vi "Analysis_Result_To_Table_Value.vi"(9 "AnalysisResults":variant[](array[variant]), 11 "All ROI":T8[](array[typedef])) -> (2 "TableValues":string[](array[string]))   [LabVIEW 2019]
uses:
  Analysis/Controls/Parttern Match/Analysis_PatternMatch_Parameter.ctl
  Analysis/Controls/Edge Detection/Analysis_Edge Detection_Parameter.ctl
  Analysis/Controls/Barcode 1D/Analysis_Barcode 1D_Parameter.ctl
  <vilib>/vision/Instrument.llb/QR Code Model Type.ctl
  <vilib>/vision/Instrument.llb/Data Matrix Polarity.ctl
  <vilib>/vision/Instrument.llb/QR Code Description Options.ctl
  <vilib>/vision/Instrument.llb/Cell Filter Mode.ctl
  <vilib>/vision/Instrument.llb/Cell Sample Size.ctl
  <vilib>/vision/Instrument.llb/Demodulation Mode.ctl
  <vilib>/vision/Instrument.llb/QR Code Search Options.ctl
  Analysis/Controls/Barcode 2D/Analysis_Barcode 2D_Parameter.ctl
  Analysis/Controls/Clamp/Analysis_Clamp_Parameter.ctl
  Analysis/Controls/Clamp MAX/Analysis_Clamp MAX_Parameter.ctl
  Analysis/Controls/Particle/Analysis_Particle_Parameter.ctl
  Analysis/Controls/Find Straight Edge/Analysis_Find Straight Edge_Parameter.ctl
  <vilib>/vision/Measure.llb/Straight Edge Process.ctl
  <vilib>/vision/Measure.llb/Straight Edge Options.ctl
  <vilib>/vision/Measure.llb/Edge Polarity.ctl
  <vilib>/vision/Measure.llb/Edge Options.ctl
  <vilib>/vision/Instrument.llb/Data Matrix Search Options.ctl
  <vilib>/vision/Instrument.llb/Data Matrix Mirror.ctl
  <vilib>/vision/Instrument.llb/Cell Fill Percentage.ctl
  <vilib>/vision/Instrument.llb/ECC Type.ctl
  <vilib>/vision/Instrument.llb/Data Matrix Description Options.ctl
  Analysis/Controls/Histogram/Analysis_Histogram_Parameter.ctl
  Analysis/Controls/Circle/Analysis_Circle_Parameter.ctl
  Analysis/Controls/Parttern Match/Analysis_PatternMatch_ResultWithnumber.ctl
  Analysis/Controls/ShapeDectect/Analysis_ShapeDectect_Parameter.ctl
  Analysis/Controls/Contour/Analysis_Contour_Result.ctl
  Analysis/Controls/ColorMatch/Analysis_ColorMatch_Result.ctl
  <vilib>/vision/Instrument.llb/Data Matrix Advanced Options.ctl
  <vilib>/vision/Instrument.llb/Data Matrix Size Options.ctl
  Process/Controls/Process_Setting.ctl
  Analysis/Controls/Analysis_Setting.ctl
  Controls/Vision_DataEntry.ctl
  <vilib>/vision/Measure.llb/Edge New.ctl
  Analysis/Controls/V_Analysis_Type.ctl
  Ctrl/VisionProcessName.ctl
panel:
  in  "output cluster 2":T1
  in  "Particle Cluster":T2
  in  "output cluster":T3
  in  "Clamp Cluster":T4={"Points"=[], "Perpendicular Lines"=[], "appended array"=[], "Line Coordinates"=[], "Clamp Settings"={"Contrast"=0, "Filter width"=0, "Steepness"=0, "Subsampling Ratio"=0, "Show Search Area"=FALSE, "Show Search Lines"=FALSE, "Show Edges Found"=FALSE, "Show Result"=FALSE}, "ROI Descriptor"={"Global Rectangle"=[], "Contours"=[]}, "Distance"=0.0, "Edge Coordinates"=[{"X"=441.67966, "Y"=663.0}, {"X"=684.4586, "Y"=655.0}], "Edge Coordinates  (Real World)"=[{"X"=441.67966, "Y"=663.0}, {"X"=684.4586, "Y"=655.0}], "Distance (Real World)"=0.0}
  in  "Edge Detection Cluster":T6 {"Edge Information"."Distance (Real-World)" format="%.2f"; "Edge Information"."Location (Real-World)"."Y" format="%.2g"; "Edge Information"."Location (Real-World)"."X" format="%.2f"; "Edge Information"."Noise" format="%.2f"; "Edge Information"."Location (Pixel)"."Y" format="%.2g"; "Edge Information"."Location (Pixel)"."X" format="%.2f"; "Edge Information"."Strength" format="%.2f"; "Edge Information"."Distance (Pixel)" format="%.2f"}
  in  "Straight Edge Cluster Array":T7(array[cluster])
  in  "Barcode 2D Result cluster":T13
  in  "Barcode 1D output cluster":T14
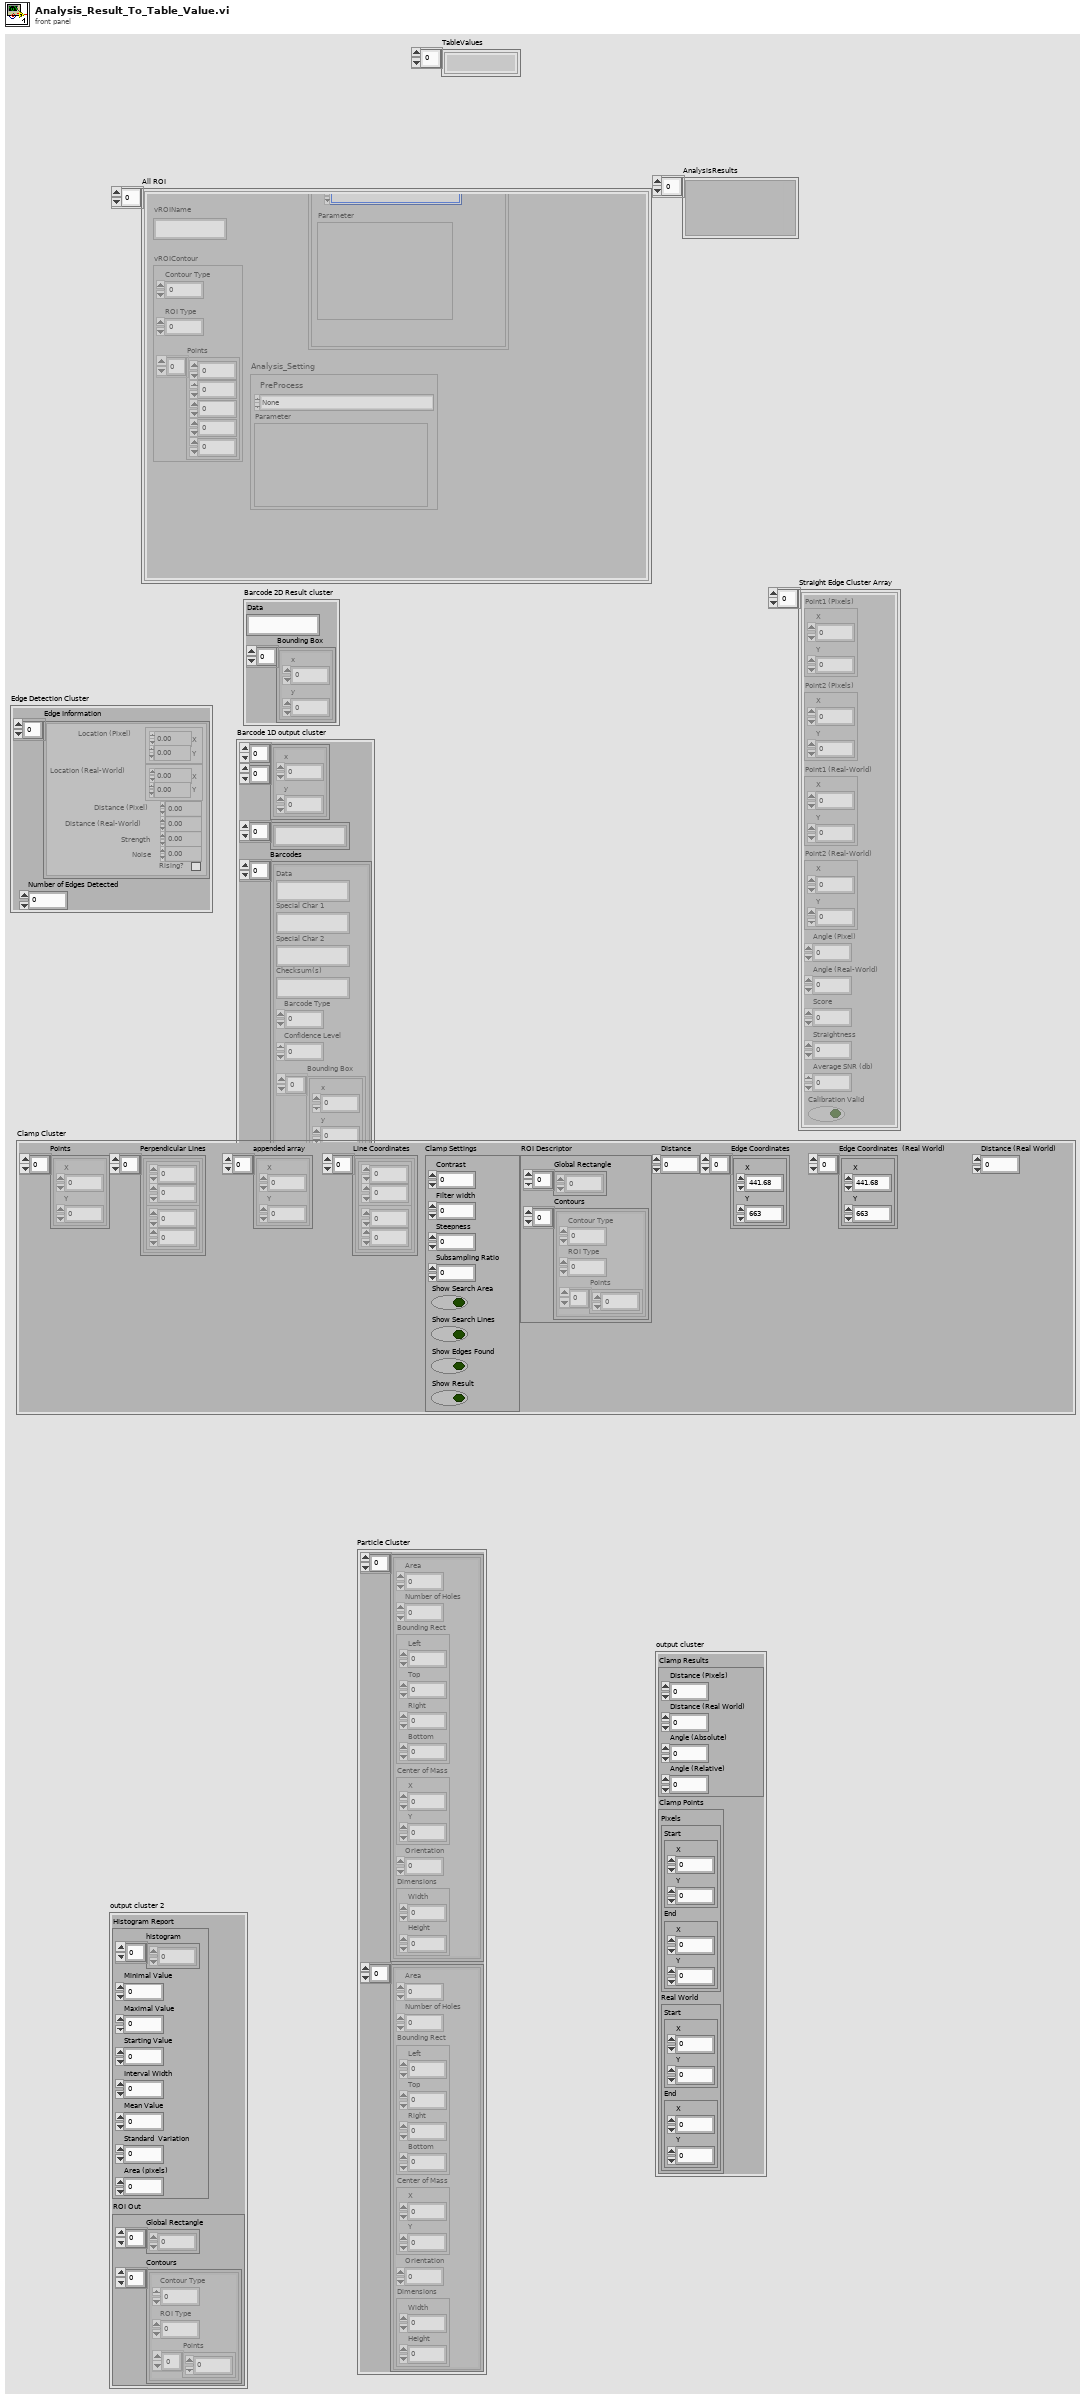
[diagram p1: front panel]
types:
  T1 = cluster{"Histogram Report":cluster{"histogram":u32[], "Minimal Value":sgl, "Maximal Value":sgl, "Starting Value":sgl, "Interval Width":sgl, "Mean Value":sgl, "Standard  Variation":sgl, "Area (pixels)":i32}, "ROI Out":cluster{"Global Rectangle":i32[], "Contours":cluster{"Contour Type":u32, "ROI Type":u32, "Points":i32[]}[]}}
  T2 = cluster{cluster{"Area":dbl, "Number of Holes":dbl, "Bounding Rect":cluster{"Left":dbl, "Top":dbl, "Right":dbl, "Bottom":dbl}, "Center of Mass":cluster{"X":dbl, "Y":dbl}, "Orientation":dbl, "Dimensions":cluster{"Width":dbl, "Height":dbl}}[], cluster{"Area":dbl, "Number of Holes":dbl, "Bounding Rect":cluster{"Left":dbl, "Top":dbl, "Right":dbl, "Bottom":dbl}, "Center of Mass":cluster{"X":dbl, "Y":dbl}, "Orientation":dbl, "Dimensions":cluster{"Width":dbl, "Height":dbl}}[]}
  T3 = cluster{"Clamp Results":cluster{"Distance (Pixels)":dbl, "Distance (Real World)":dbl, "Angle (Absolute)":dbl, "Angle (Relative)":dbl}, "Clamp Points":cluster{"Pixels ":cluster{"Start":cluster{"X":dbl, "Y":dbl}, "End":cluster{"X":dbl, "Y":dbl}}, "Real World":cluster{"Start":cluster{"X":dbl, "Y":dbl}, "End":cluster{"X":dbl, "Y":dbl}}}}
  T4 = cluster{"Points":cluster{"X":sgl, "Y":sgl}[], "Perpendicular Lines":cluster{cluster{sgl, sgl}, cluster{sgl, sgl}}[], "appended array":cluster{"X":sgl, "Y":sgl}[], "Line Coordinates":cluster{cluster{sgl, sgl}, cluster{sgl, sgl}}[], "Clamp Settings":cluster{"Contrast":i32, "Filter width":i32, "Steepness":i32, "Subsampling Ratio":u32, "Show Search Area":bool, "Show Search Lines":bool, "Show Edges Found":bool, "Show Result":bool}, "ROI Descriptor":cluster{"Global Rectangle":i32[], "Contours":cluster{"Contour Type":u32, "ROI Type":u32, "Points":i32[]}[]}, "Distance":sgl, "Edge Coordinates":cluster{"X":sgl, "Y":sgl}[], "Edge Coordinates  (Real World)":cluster{"X":sgl, "Y":sgl}[], "Distance (Real World)":sgl}
  T5 = typedef "Edge New.ctl" = cluster{"Location (Pixel)":cluster{"X":sgl, "Y":sgl}, "Location (Real-World)":cluster{"X":sgl, "Y":sgl}, "Distance (Pixel)":dbl, "Distance (Real-World)":dbl, "Strength":dbl, "Noise":dbl, "Rising?":bool}
  T6 = cluster{"Edge Information":T5[], "Number of Edges Detected":i32}
  T7 = cluster{"Point1 (Pixels)":cluster{"X":sgl, "Y":sgl}, "Point2 (Pixels)":cluster{"X":sgl, "Y":sgl}, "Point1 (Real-World)":cluster{"X":sgl, "Y":sgl}, "Point2 (Real-World)":cluster{"X":sgl, "Y":sgl}, "Angle (Pixel)":dbl, "Angle (Real-World)":dbl, "Score":dbl, "Straightness":dbl, "Average SNR (db)":dbl, "Calibration Valid":bool}[]
  T8 = typedef "Vision_DataEntry.ctl" = cluster{"vROIName":string, "vROIContour":cluster{"Contour Type":u32, "ROI Type":u32, "Points":i32[]}, "ProcessSetting":T9[], "Analysis_Setting":T11}
  T9 = typedef "Process_Setting.ctl" = cluster{"Enum_PreProcess":T10, "Parameter":string}
  T10 = typedef "VisionProcessName.ctl" = enum16{"*CamParameter*", "CamAttributes", "*Preprocess*", "CG_Brightness", "C_Plane Extraction", "C_Threshold", "G_Lookup Table", "G_Threshold"}
  T11 = typedef "Analysis_Setting.ctl" = cluster{"PreProcess":T12, "Parameter":string}
  T12 = typedef "V_Analysis_Type.ctl" = enum16{"None", "C_Color Pattern Matching", "G_PatternMatching", "G_ShapeDectect", "G_GeometricMatch", "B_Area Check"}
  T13 = cluster{"Data":string, "Bounding Box":cluster{"x":sgl, "y":sgl}[]}
  T14 = cluster{cluster{"x":sgl, "y":sgl}[][], string[], "Barcodes":cluster{"Data":string, "Special Char 1":string, "Special Char 2":string, "Checksum(s)":string, "Barcode Type":u32, "Confidence Level":sgl, "Bounding Box":cluster{"x":sgl, "y":sgl}[]}[]}
  T15 = typedef "ROI Descriptor" = cluster{"Global Rectangle":i32[], "Contours":cluster{"ID":enum32{"External", "Internal"}, "Type":u32, "Coordinates":i32[]}[]}
  T16 = cluster{"Algorithm":i32, "Match Parameters":cluster{"Number of Matches Requested":i32, "Minimum Match Score":sgl, "Angle Ranges":cluster{"Start Angle":sgl, "End Angle":sgl}[]}, "ROI Descriptor":T15, "Advanced Options":cluster{"Item":u16, "Value":dbl}[], "Template path":string}
  T17 = typedef "Analysis_Histogram_Parameter.ctl" = cluster{"Interval Range":cluster{"Minimum":sgl, "Maximum":sgl}, "ROI Out":cluster{"Global Rectangle":i32[], "Contours":cluster{"Contour Type":u32, "ROI Type":u32, "Points":i32[]}[]}, "Number of Classes":i32}
  T18 = cluster{"ROI Descriptor out":T15, "ROI Descriptor out":T15, "Fitted Circle":cluster{"Center (Pixels)":cluster{"X":sgl, "Y":sgl}, "Radius (Pixels)":dbl, "Center (Real-World)":cluster{"X":sgl, "Y":sgl}, "Radius (Real-World)":dbl, "Roundness (Real-World)":dbl, "Average Strength":dbl, "Average SNR (dB)":dbl}}
  T19 = typedef "Analysis_ShapeDectect_Parameter.ctl" = cluster{"Enum_ShapeType":enum16{"Circles", "Ellipses", "Lines", "Rectangles"}, "MaxParticle":i32, "Descriptor":cluster{"Set 1":dbl, "Set 2":dbl, "Set 3":dbl, "Set 4":dbl}, "Match Options":cluster{"Rotation":bool, "Scale":bool, "Occlusion":bool, "Range Settings":cluster{"Match Constraints":u32, "Min":dbl, "Max":dbl}[]}, "Curve Parameters":cluster{"Extraction Mode":u32, "Edge Threshold":i32, "Edge Filter Size":u32, "Min Length":i32, "Row Search Step Size":i32, "Col Search Step Size":i32, "Max Endpoint Gap":i32, "Closed":bool, "Subpixel":bool}, " score":dbl}
  T20 = typedef "Analysis_Contour_Result.ctl" = cluster{"Points (pixel)":cluster{"X":dbl, "Y":dbl}[], "Points (real)":cluster{"X":dbl, "Y":dbl}[], "Length (pixel)":dbl, "Length (real)":dbl}
  T21 = typedef "Analysis_ColorMatch_Result.ctl" = cluster{"Match Flag":bool[], "Match Score":i32[], "ROI Descriptor":T15}
  T22 = typedef "Analysis_Type.ctl" = u16
  T23 = typedef "Analysis_PatternMatch_ResultWithnumber.ctl" = cluster{"numbers":i32, "results":cluster{"ROI Descriptor out":T15, "Point":T24, "Angle":sgl, "Score":sgl, "Real World Coordinates":cluster{"X":sgl, "Y":sgl}, "Rectangle":T25}[]}
  T24 = typedef "IMAQ Point" = cluster{"X":sgl, "Y":sgl}
  T25 = typedef "IMAQ Rectangle" = cluster{"Left":i32, "Top":i32, "Right":i32, "Bottom":i32, "Rotation":dbl}
  T26 = typedef "Analysis_PatternMatch_Parameter.ctl" = cluster{"Algorithm":i32, "Match Parameters":cluster{"Number of Matches Requested":i32, "Minimum Match Score":sgl, "Angle Ranges":cluster{"Start Angle":sgl, "End Angle":sgl}[]}, "ROI Descriptor":T15, "Advanced Options":cluster{"Item":u16, "Value":dbl}[], "Template path":string, "XOffset":i32, "YOffset":i32}
  T27 = cluster{"Number of Matches Requested":i32, "Minimum Match Score":sgl, "Angle Ranges":cluster{"Start Angle":sgl, "End Angle":sgl}[]}
  T28 = typedef "Analysis_Edge Detection_Parameter.ctl" = cluster{"Edge Options":cluster{"Edge Polarity":u16, "Kernel Size":u32, "Width":u32, "Minimum Edge Strength":dbl, "Interpolation Type":u16, "Data Processing Method":u16}, "Process":u16, "Number of Matches Requested":i32, "ROI Descriptor":cluster{"Global Rectangle":i32[], "Contours":cluster{"Contour Type":u32, "ROI Type":u32, "Points":i32[]}[]}}
  T29 = typedef "Analysis_Barcode 1D_Parameter.ctl" = cluster{"Barcode Search Options":cluster{"Min Bar Width":dbl, "Min Edge Strength":dbl, "Min Bars":dbl, "Skip Location Search?":bool}, "Barcode Types To Search":enum16{"Reserved", "Codabar", "Code 39", "Code 93", "Code 128", "EAN 8", "EAN 13", "Interleaved 2 of 5", "MSI", "UPCA", "Pharmacode", "RSS Limited"}[], "Barcode Grading Options":cluster{"Calculate Grading Report":bool, "Scan Width ":dbl}, "Number of Matches Requested":i32, "ROI":cluster{"Global Rectangle":i32[], "Contours":cluster{"Contour Type":u32, "ROI Type":u32, "Points":i32[]}[]}}
  T30 = cluster{"Data":string, "Special Char 1":string, "Special Char 2":string, "Checksum(s)":string, "Barcode Type":u32, "Confidence Level":sgl, "Bounding Box":cluster{"x":sgl, "y":sgl}[]}[]
  T31 = typedef "Analysis_Barcode 2D_Parameter.ctl" = cluster{"ROI":cluster{"Global Rectangle":i32[], "Contours":cluster{"Contour Type":u32, "ROI Type":u32, "Points":i32[]}[]}, "Barcode Type":enum16{"Data Matrix", "PDF417", "QR Code"}, "Data Matrix Parameter":cluster{"Data Matrix Description Options":T32, "Data Matrix Search Options":T37, "Data Matrix Size Options":T41, "Advanced Options":T42[]}, "PDF147 Search Mode":T43, "QR Code Parameter":cluster{"QR Search Options":T44, "QR Description Options":T45, "QR Code Cell Size (pixels)":cluster{"Minimum Size":u32, "Maximum Size":u32}}}
  T32 = typedef "Data Matrix Description Options.ctl" = cluster{"Aspect Ratio":sgl, "Rows":u32, "Columns":u32, "Rectangle":bool, "ECC":T33, "Barcode Polarity":T34, "Cell Fill Percentage":T35, "Minimum Border Integrity %":sgl, "Mirror Mode":T36}
  T33 = typedef "ECC Type.ctl" = i32
  T34 = typedef "Data Matrix Polarity.ctl" = i32
  T35 = typedef "Cell Fill Percentage.ctl" = i32
  T36 = typedef "Data Matrix Mirror.ctl" = i32
  T37 = typedef "Data Matrix Search Options.ctl" = cluster{"Rotation Mode":enum32{"Unlimited", "0 Degrees", "90 Degrees", "180 Degrees", "270 Degrees"}, "Skip Location?":bool, "Edge Threshold":u32, "Demodulation Mode":T38, "Cell Sample Size":T39, "Cell Filter Mode":T40, "Skew Degrees Allowed":u32, "Maximum Iterations":u32, "Initial Search Vector Width":u32}
  T38 = typedef "Demodulation Mode.ctl" = i32
  T39 = typedef "Cell Sample Size.ctl" = i32
  T40 = typedef "Cell Filter Mode.ctl" = i32
  T41 = typedef "Data Matrix Size Options.ctl" = cluster{"Data Matrix Size":cluster{"Minimum Size":u32, "Maximum Size":u32}, "Quiet Zone Width":u32}
  T42 = typedef "Data Matrix Advanced Options.ctl" = cluster{"Option":enum32{"Line Detection", "HighLight Filter", "Aggressive", "FNC1", "Refine Bounding Box"}, " Value":dbl}
  T43 = typedef "PDF417 Search Mode" = enum32{"Multiple Barcodes", "Single Barcode, Conservative"}
  T44 = typedef "QR Code Search Options.ctl" = cluster{"Rotation Mode":enum32{"Unlimited", "0 Degrees", "90 Degrees", "180 Degrees", "270 Degrees"}, "Skip Location?":bool, "Edge Threshold":u32, "Demodulation Mode":T38, "Cell Sample Size":T39, "Cell Filter Mode":T40, "Skew Degrees Allowed":u32}
  T45 = typedef "QR Code Description Options.ctl" = cluster{"Matrix Size (cells)":i32, "Barcode Polarity":T34, "Mirror Mode":i32, "QR Model":T46}
  T46 = typedef "QR Code Model Type.ctl" = i32
  T47 = typedef "Analysis_Clamp_Parameter.ctl" = cluster{"Clamp Settings":cluster{"Contrast":i32, "Filter width":i32, "Steepness":i32, "Subsampling Ratio":u32, "Show Search Area":bool, "Show Search Lines":bool, "Show Edges Found":bool, "Show Result":bool}, "ROI Descriptor":cluster{"Global Rectangle":i32[], "Contours":cluster{"Contour Type":u32, "ROI Type":u32, "Points":i32[]}[]}, "Process":u16}
  T48 = typedef "Analysis_Clamp MAX_Parameter.ctl" = cluster{"Overlay Settings":cluster{"Show Search Area":bool, "Show Curves":bool, "Show Clamp Locations":bool, "Show Result":bool, "Search Area Color":u32, "Curves Color":u32, "Clamp Locations Color":u32, "Result Color":u32, "Overlay Group Name":string}, "Curve Extraction Settings":cluster{"Extraction Mode":u32, "Edge Threshold":i32, "Edge Filter Size":u32, "Min Length":i32, "Row Search Step Size":i32, "Col Search Step Size":i32, "Max Endpoint Gap":i32, "Closed":bool, "Subpixel":bool}, "Clamp Settings":cluster{"Angle Range (+/-)":dbl, "Edge Polarity":cluster{"Start":u32, "End":u32}}, "ROI":cluster{"Global Rectangle":i32[], "Contours":cluster{"Contour Type":u32, "ROI Type":u32, "Points":i32[]}[]}}
  T49 = typedef "Analysis_Particle_Parameter.ctl" = cluster{"Selected Particle":i32, "Connectivity 4/8 (8)":bool, "MaxParticle":i32}
  T50 = typedef "Analysis_Find Straight Edge_Parameter.ctl" = cluster{"ROI Descriptor":cluster{"Global Rectangle":i32[], "Contours":cluster{"Contour Type":u32, "ROI Type":u32, "Points":i32[]}[]}, "Number of Matches Requested":i32, "Edge Info Size":i32, "Options":cluster{"Search Direction":u32, "Edge Options":T51, "Show Search Area":bool, "Show Search Lines":bool, "Show Edges Found":bool, "Show Result":bool, "Search Area Color":u32, "Search Lines Color":u32, "Edge Locations Color":u32, "Result Color":u32, "Overlay Group Name":string}, "Line Fit Options":T53}
  T51 = typedef "Edge Options.ctl" = cluster{"Edge Polarity":T52, "Kernel Size":u32, "Width":u32, "Minimum Edge Strength":sgl, "Interpolation Type":enum32{"Zero Order", "Bilinear", "Quadratic", "Cubic", "Bilinear Fixed"}, "Data Processing Method":enum32{"Average", "Median"}}
  T52 = typedef "Edge Polarity.ctl" = u32
  T53 = typedef "Straight Edge Options.ctl" = cluster{"Number of Lines":i32, "Type":T54, "Min. Score":dbl, "Max. Score":dbl, "Orientation":dbl, "Angle Range":dbl, "Angle Tolerance":dbl, "Step Size":u32, "Min. SNR (db)":dbl, "Min. Points (%)":dbl, "Hough Iterations":i32}
  T54 = typedef "Straight Edge Process.ctl" = enum32{"First Edge Rake", "Best Edge Rake", "Hough Edge Rake", "First Edge Projection", "Best Edge Projection"}
  T55 = typedef "Analysis_Circle_Parameter.ctl" = cluster{"ROI Descriptor":cluster{"Global Rectangle":i32[], "Contours":cluster{"Contour Type":u32, "ROI Type":u32, "Points":i32[]}[]}, "Options":cluster{"Search  Direction":u32, "Edge Options":T51, "Show Search Area":bool, "Show Search Lines":bool, "Show Edges Found":bool, "Show Result":bool, "Search Area Color":u32, "Search Lines Color":u32, "Edge Locations Color":u32, "Result Color":u32, "Overlay Group Name":string}, "Circle Fit Options":cluster{"Process":enum16{"Get First Edge", "Get First + Last Edge", "Get All Edges", "Get Best Edge"}, "Step Size":dbl, "Max Pixel Radius":i32}}
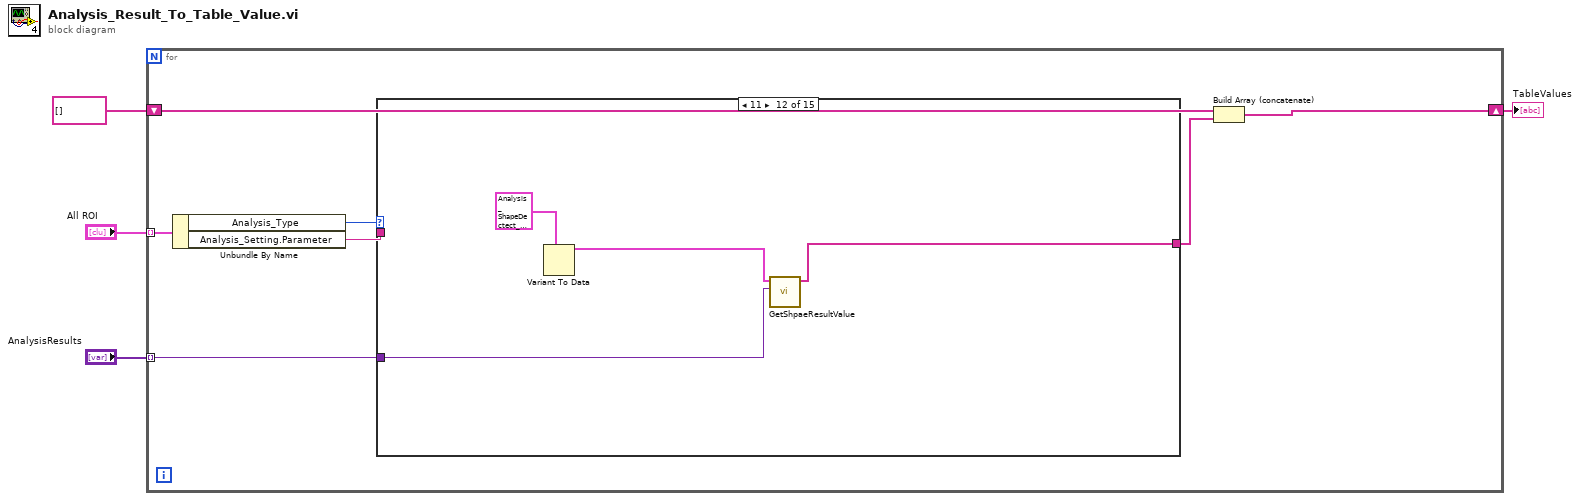
[diagram p0: block diagram]
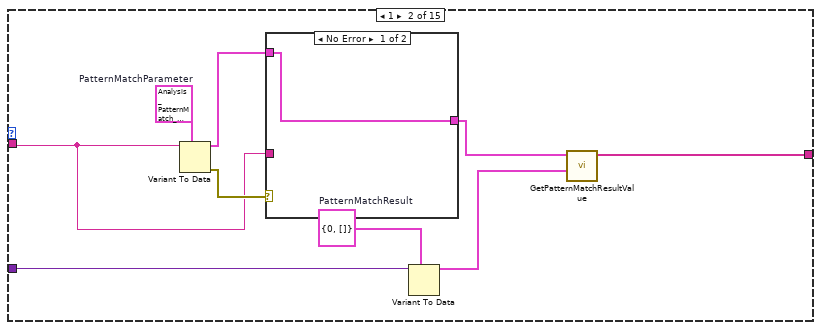
[diagram p3: hidden frame]
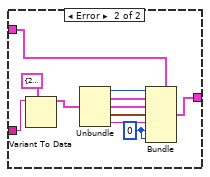
[diagram p4: hidden frame]
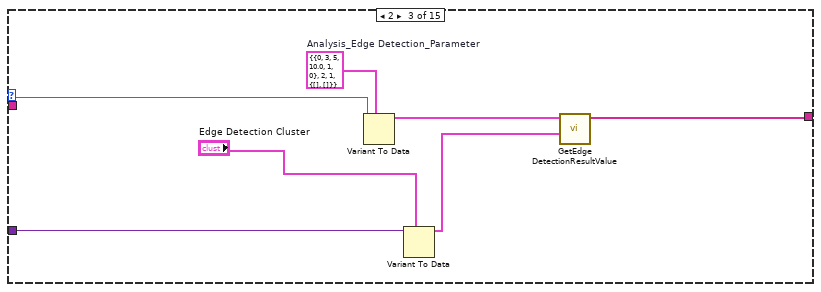
[diagram p5: hidden frame]
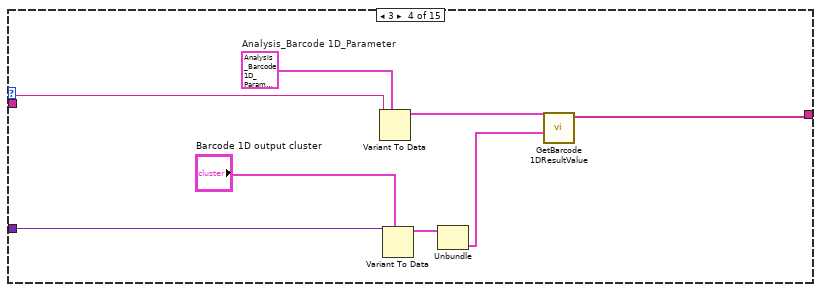
[diagram p6: hidden frame]
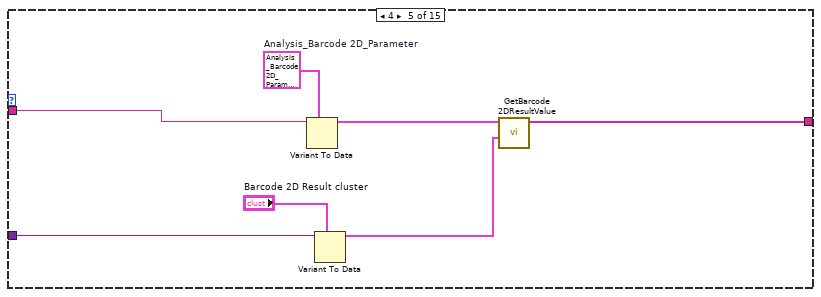
[diagram p7: hidden frame]
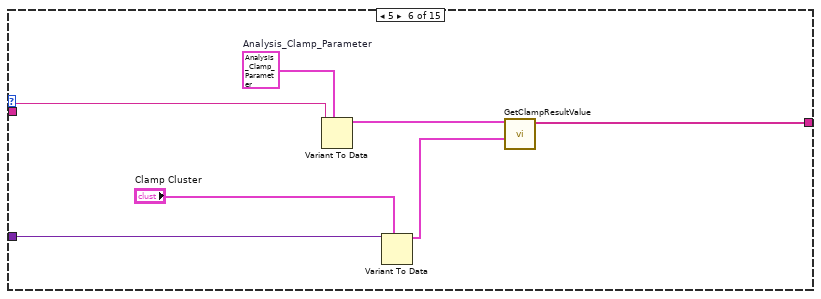
[diagram p8: hidden frame]
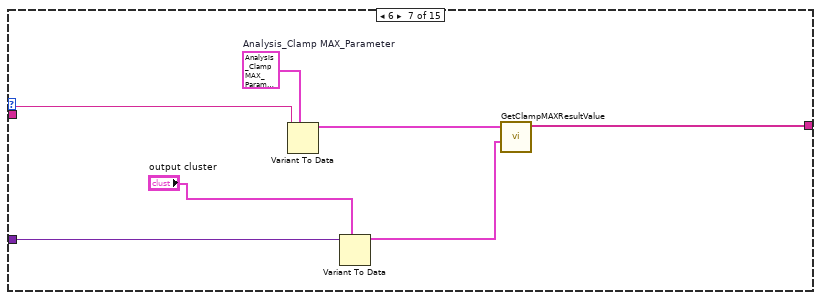
[diagram p9: hidden frame]
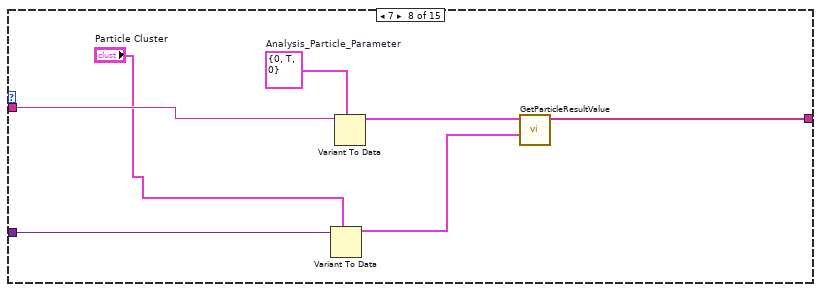
[diagram p10: hidden frame]
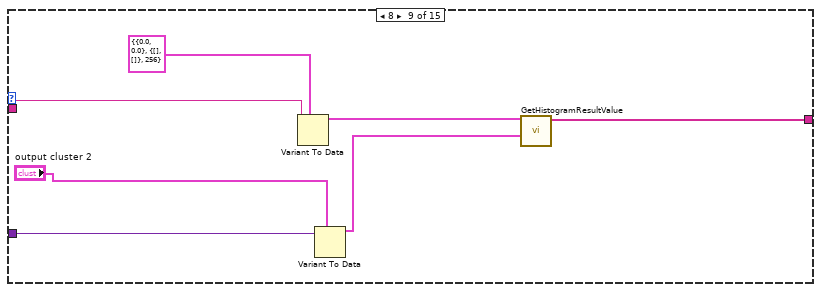
[diagram p11: hidden frame]
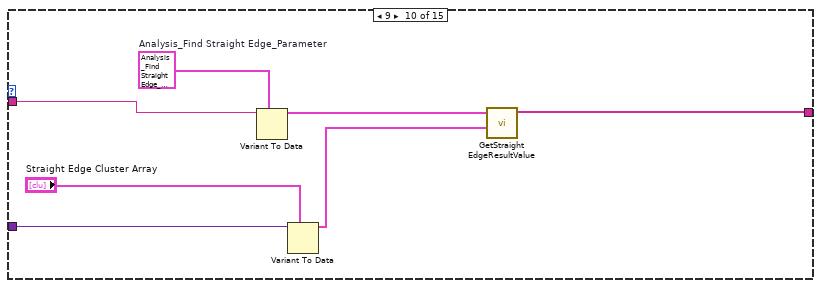
[diagram p12: hidden frame]
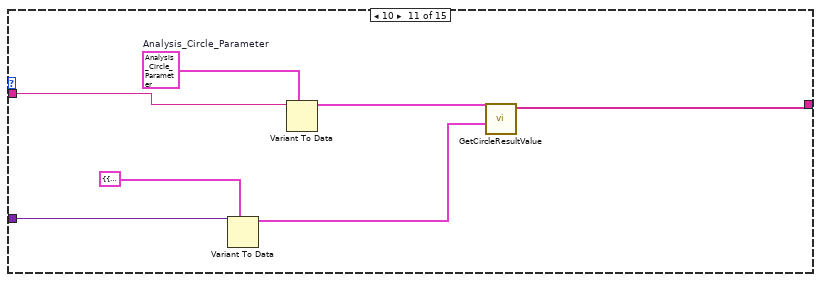
[diagram p13: hidden frame]
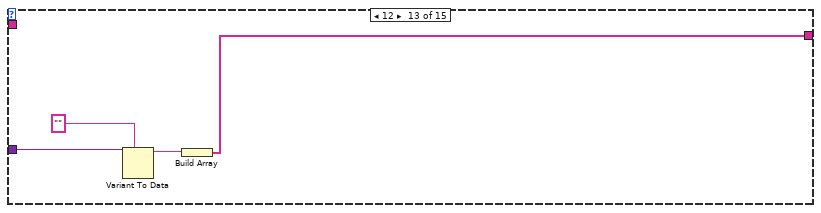
[diagram p14: hidden frame]
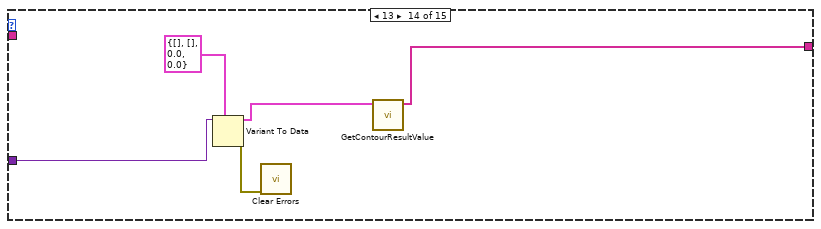
[diagram p15: hidden frame]
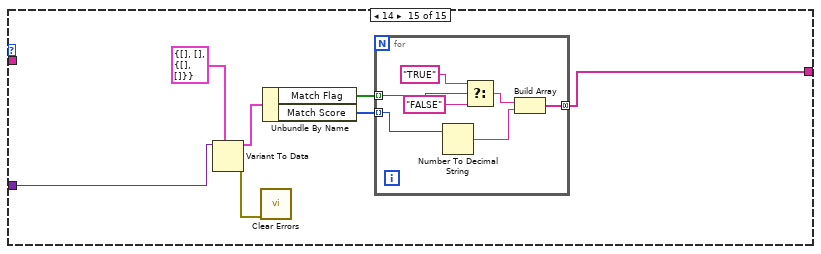
[diagram p16: hidden frame]
diagram:
  n1 = for {
    tunnel: "All ROI" -> [w11] mode=indexing
    shift-right: [w7] -> w1
    shift-left: string[] [] -> [w8]
    tunnel: "AnalysisResults" -> [w5] mode=indexing
    n2 = Unbundle By Name(w11) -> ("Analysis_Type"=w10:T22, "Analysis_Setting.Parameter"=w9:string)
    n3 = case shown="11" w10 {
      tunnel: w9 -> [_ w13 w39 w46 w52 w60 w68 w75 w82 w89 w96 _ _ _ _]
      tunnel: [_ w19 w36 w44 w48 w59 w65 w71 w80 w86 w92 w97 w101 w105 w110] -> w6
      tunnel: w5 -> [_ w18 w35 w47 w54 w61 w67 w74 w81 w88 w95 w98 w104 w108 w116]
      frame 0, Default {
      }
      frame 1 {
        w16 = T23 {"numbers"=0, "results"=[]}  # PatternMatchResult
        w20 = T26 {"Algorithm"=2, "Match Parameters"={"Number of Matches Requested"=1, "Minimum Match Score"=750.0, "Angle Ranges"=[]}, "ROI Descriptor"={"Global Rectangle"=[], "Contours"=[]}, "Advanced Options"=[{"Item"=1, "Value"=1.0}, {"Item"=103, "Value"=1.0}], "Template path"="", "XOffset"=0, "YOffset"=0}  # PatternMatchParameter
        n4 = Variant To Data(type=w20, Variant=w13) -> (data=w14:T26, error out=w15:errorcluster)  [unwired: 1 in]
        n5 = case shown="No Error" w15 {
          tunnel: w13 -> [_ w31]
          tunnel: [w21 w29] -> w12
          tunnel: w14 -> [w21 w30]
          frame No Error {
          }
          frame Error {
            w22 = 0 ("XOffset")
            n6 = Variant To Data(type=T16 {"Algorithm"=2, "Match Parameters"={"Number of Matches Requested"=1, "Minimum Match Score"=750.0, "Angle Ranges"=[]}, "ROI Descriptor"={"Global Rectangle"=[], "Contours"=[]}, "Advanced Options"=[{"Item"=1, "Value"=1.0}, {"Item"=103, "Value"=1.0}], "Template path"=""} ("PatternMatchParameter"), Variant=w31) -> (data=w28:T16)  [unwired: 1 in, 1 out]
            n7 = Unbundle(w28) -> ("Algorithm"=w27:i32, "Match Parameters"=w26:T27, "ROI Descriptor"=w25:T15, "Advanced Options"=w24:cluster{"Item":u16, "Value":dbl}[], "Template path"=w23:string)
            n8 = Bundle(cluster=w30, "Algorithm"=w27, "Match Parameters"=w26, "ROI Descriptor"=w25, "Advanced Options"=w24, "Template path"=w23, "XOffset"=w22, "YOffset"=w22) -> (w29:T26)
          }
        }
        n9 = Variant To Data(type=w16, Variant=w18) -> (data=w17:T23)  [unwired: 1 in, 1 out]
        n10 = call "GetPatternMatchResultValue.vi"("PatternMatchResult"=w17, "PatternMatchParameter"=w12) -> ("ResultValues"=w19:string[])  [unwired: 8 in, 1 out]
      }
      frame 2 {
        w38 = T28 {"Edge Options"={"Edge Polarity"=0, "Kernel Size"=3, "Width"=5, "Minimum Edge Strength"=10.0, "Interpolation Type"=1, "Data Processing Method"=0}, "Process"=2, "Number of Matches Requested"=1, "ROI Descriptor"={"Global Rectangle"=[], "Contours"=[]}}  # Analysis_Edge Detection_Parameter
        n11 = Variant To Data(type=w38, Variant=w39) -> (data=w37:T28)  [unwired: 1 in, 1 out]
        n12 = Variant To Data(type="Edge Detection Cluster", Variant=w35) -> (data=w34:T6)  [unwired: 1 in, 1 out]
        n13 = call "GetEdge DetectionResultValue.vi"("data"=w34, "Analysis_Edge Detection_Parameter"=w37) -> ("ResultValues"=w36:string[])  [unwired: 8 in, 1 out]
      }
      frame 3 {
        w45 = T29 {"Barcode Search Options"={"Min Bar Width"=0.0, "Min Edge Strength"=0.0, "Min Bars"=0.0, "Skip Location Search?"=FALSE}, "Barcode Types To Search"=[enum."EAN 13", enum."Code 128", enum."Code 39"], "Barcode Grading Options"={"Calculate Grading Report"=FALSE, "Scan Width "=0.0}, "Number of Matches Requested"=1, "ROI"={"Global Rectangle"=[], "Contours"=[]}}  # Analysis_Barcode 1D_Parameter
        n14 = Variant To Data(type=w45, Variant=w46) -> (data=w43:T29)  [unwired: 1 in, 1 out]
        n15 = Variant To Data(type="Barcode 1D output cluster", Variant=w47) -> (data=w41:T14)  [unwired: 1 in, 1 out]
        n16 = Unbundle(w41) -> ("Barcodes"=w40:T30)  [unwired: 2 out]
        n17 = call "GetBarcode 1DResultValue.vi"("data"=w40, "Analysis_Barcode 1D_Parameter"=w43) -> ("ResultValues"=w44:string[])  [unwired: 8 in, 1 out]
      }
      frame 4 {
        w51 = T31 {"ROI"={"Global Rectangle"=[], "Contours"=[]}, "Barcode Type"=enum."PDF417", "Data Matrix Parameter"={"Data Matrix Description Options"={"Aspect Ratio"=0.0, "Rows"=0, "Columns"=0, "Rectangle"=FALSE, "ECC"=-2, "Barcode Polarity"=0, "Cell Fill Percentage"=-2, "Minimum Border Integrity %"=80.0, "Mirror Mode"=-2}, "Data Matrix Search Options"={"Rotation Mode"=enum."Unlimited", "Skip Location?"=FALSE, "Edge Threshold"=30, "Demodulation Mode"=-2, "Cell Sample Size"=-2, "Cell Filter Mode"=-2, "Skew Degrees Allowed"=5, "Maximum Iterations"=500, "Initial Search Vector Width"=5}, "Data Matrix Size Options"={"Data Matrix Size"={"Minimum Size"=0, "Maximum Size"=0}, "Quiet Zone Width"=10}, "Advanced Options"=[]}, "PDF147 Search Mode"=enum."Multiple Barcodes", "QR Code Parameter"={"QR Search Options"={"Rotation Mode"=enum."Unlimited", "Skip Location?"=FALSE, "Edge Threshold"=30, "Demodulation Mode"=-2, "Cell Sample Size"=-2, "Cell Filter Mode"=-2, "Skew Degrees Allowed"=5}, "QR Description Options"={"Matrix Size (cells)"=0, "Barcode Polarity"=-2, "Mirror Mode"=-2, "QR Model"=0}, "QR Code Cell Size (pixels)"={"Minimum Size"=3, "Maximum Size"=7}}}  # Analysis_Barcode 2D_Parameter
        n18 = Variant To Data(type=w51, Variant=w52) -> (data=w50:T31)  [unwired: 1 in, 1 out]
        n19 = Variant To Data(type="Barcode 2D Result cluster", Variant=w54) -> (data=w49:T13)  [unwired: 1 in, 1 out]
        n20 = call "GetBarcode 2DResultValue.vi"("data"=w49, "Analysis_Barcode 2D_Parameter"=w50) -> ("ResultValues"=w48:string[])  [unwired: 8 in, 1 out]
      }
      frame 5 {
        w58 = T47 {"Clamp Settings"={"Contrast"=40, "Filter width"=4, "Steepness"=2, "Subsampling Ratio"=5, "Show Search Area"=TRUE, "Show Search Lines"=TRUE, "Show Edges Found"=TRUE, "Show Result"=TRUE}, "ROI Descriptor"={"Global Rectangle"=[498, 111, 1545, 770], "Contours"=[{"Contour Type"=0, "ROI Type"=12, "Points"=[498, 111, 1545, 770, 0]}]}, "Process"=0}  # Analysis_Clamp_Parameter
        n21 = Variant To Data(type=w58, Variant=w60) -> (data=w57:T47)  [unwired: 1 in, 1 out]
        n22 = Variant To Data(type="Clamp Cluster", Variant=w61) -> (data=w56:T4)  [unwired: 1 in, 1 out]
        n23 = call "GetClampResultValue.vi"("data"=w56, "Analysis_Clamp_Parameter"=w57) -> ("ResultValues"=w59:string[])  [unwired: 8 in, 1 out]
      }
      frame 6 {
        w66 = T48 {"Overlay Settings"={"Show Search Area"=FALSE, "Show Curves"=FALSE, "Show Clamp Locations"=FALSE, "Show Result"=FALSE, "Search Area Color"=0, "Curves Color"=0, "Clamp Locations Color"=0, "Result Color"=0, "Overlay Group Name"=""}, "Curve Extraction Settings"={"Extraction Mode"=0, "Edge Threshold"=0, "Edge Filter Size"=0, "Min Length"=0, "Row Search Step Size"=0, "Col Search Step Size"=0, "Max Endpoint Gap"=0, "Closed"=FALSE, "Subpixel"=FALSE}, "Clamp Settings"={"Angle Range (+/-)"=0.0, "Edge Polarity"={"Start"=0, "End"=0}}, "ROI"={"Global Rectangle"=[], "Contours"=[]}}  # Analysis_Clamp MAX_Parameter
        n24 = Variant To Data(type=w66, Variant=w68) -> (data=w64:T48)  [unwired: 1 in, 1 out]
        n25 = Variant To Data(type="output cluster", Variant=w67) -> (data=w62:T3)  [unwired: 1 in, 1 out]
        n26 = call "GetClampMAXResultValue.vi"("data"=w62, "Analysis_Clamp MAX_Parameter"=w64) -> ("ResultValues"=w65:string[])  [unwired: 8 in, 1 out]
      }
      frame 7 {
        w73 = T49 {"Selected Particle"=0, "Connectivity 4/8 (8)"=TRUE, "MaxParticle"=0}  # Analysis_Particle_Parameter
        n27 = Variant To Data(type="Particle Cluster", Variant=w74) -> (data=w70:T2)  [unwired: 1 in, 1 out]
        n28 = Variant To Data(type=w73, Variant=w75) -> (data=w72:T49)  [unwired: 1 in, 1 out]
        n29 = call "GetParticleResultValue.vi"("Data"=w70, "Analysis_Particle_Parameter"=w72) -> ("ResultValues"=w71:string[])  [unwired: 8 in, 1 out]
      }
      frame 8 {
        n30 = Variant To Data(type=T17 {"Interval Range"={"Minimum"=0.0, "Maximum"=0.0}, "ROI Out"={"Global Rectangle"=[], "Contours"=[]}, "Number of Classes"=256} ("Analysis_Histogram_Parameter"), Variant=w82) -> (data=w79:T17)  [unwired: 1 in, 1 out]
        n31 = Variant To Data(type="output cluster 2", Variant=w81) -> (data=w76:T1)  [unwired: 1 in, 1 out]
        n32 = call "GetHistogramResultValue.vi"("data"=w76, "Analysis_Histogram_Parameter"=w79) -> ("ResultValues"=w80:string[])  [unwired: 8 in, 1 out]
      }
      frame 9 {
        w87 = T50 {"ROI Descriptor"={"Global Rectangle"=[], "Contours"=[]}, "Number of Matches Requested"=4, "Edge Info Size"=0, "Options"={"Search Direction"=0, "Edge Options"={"Edge Polarity"=0, "Kernel Size"=4, "Width"=3, "Minimum Edge Strength"=1024.0, "Interpolation Type"=enum."Zero Order", "Data Processing Method"=enum."Median"}, "Show Search Area"=FALSE, "Show Search Lines"=FALSE, "Show Edges Found"=FALSE, "Show Result"=TRUE, "Search Area Color"=5, "Search Lines Color"=3, "Edge Locations Color"=50, "Result Color"=1, "Overlay Group Name"=""}, "Line Fit Options"={"Number of Lines"=0, "Type"=enum."Best Edge Rake", "Min. Score"=0.0, "Max. Score"=25.0, "Orientation"=5.0, "Angle Range"=45.0, "Angle Tolerance"=1.0, "Step Size"=7, "Min. SNR (db)"=0.0, "Min. Points (%)"=25.0, "Hough Iterations"=5}}  # Analysis_Find Straight Edge_Parameter
        n33 = Variant To Data(type=w87, Variant=w89) -> (data=w85:T50)  [unwired: 1 in, 1 out]
        n34 = Variant To Data(type="Straight Edge Cluster Array", Variant=w88) -> (data=w83:T7)  [unwired: 1 in, 1 out]
        n35 = call "GetStraight EdgeResultValue.vi"("data"=w83, "Analysis_Find Straight Edge_Parameter"=w85) -> ("ResultValues"=w86:string[])  [unwired: 8 in, 1 out]
      }
      frame 10 {
        w94 = T55 {"ROI Descriptor"={"Global Rectangle"=[], "Contours"=[]}, "Options"={"Search  Direction"=0, "Edge Options"={"Edge Polarity"=0, "Kernel Size"=3, "Width"=3, "Minimum Edge Strength"=10.0, "Interpolation Type"=enum."Bilinear Fixed", "Data Processing Method"=enum."Average"}, "Show Search Area"=FALSE, "Show Search Lines"=FALSE, "Show Edges Found"=FALSE, "Show Result"=TRUE, "Search Area Color"=65280, "Search Lines Color"=255, "Edge Locations Color"=16776960, "Result Color"=16711680, "Overlay Group Name"=""}, "Circle Fit Options"={"Process"=enum."Get First Edge", "Step Size"=3.0, "Max Pixel Radius"=3}}  # Analysis_Circle_Parameter
        n36 = Variant To Data(type=T18 {"ROI Descriptor out"={"Global Rectangle"=[], "Contours"=[]}, "ROI Descriptor out"={"Global Rectangle"=[], "Contours"=[]}, "Fitted Circle"={"Center (Pixels)"={"X"=0.0, "Y"=0.0}, "Radius (Pixels)"=0.0, "Center (Real-World)"={"X"=0.0, "Y"=0.0}, "Radius (Real-World)"=0.0, "Roundness (Real-World)"=0.0, "Average Strength"=0.0, "Average SNR (dB)"=0.0}} ("output cluster"), Variant=w95) -> (data=w90:T18)  [unwired: 1 in, 1 out]
        n37 = Variant To Data(type=w94, Variant=w96) -> (data=w93:T55)  [unwired: 1 in, 1 out]
        n38 = call "GetCircleResultValue.vi"("data"=w90, "Analysis_Circle_Parameter"=w93) -> ("ResultValues"=w92:string[])  [unwired: 8 in, 1 out]
      }
      frame 11 {
        n39 = Variant To Data(type=T19 {"Enum_ShapeType"=enum."Circles", "MaxParticle"=1, "Descriptor"={"Set 1"=100.0, "Set 2"=10.0, "Set 3"=200.0, "Set 4"=10.0}, "Match Options"={"Rotation"=TRUE, "Scale"=FALSE, "Occlusion"=FALSE, "Range Settings"=[{"Match Constraints"=0, "Min"=0.0, "Max"=360.0}]}, "Curve Parameters"={"Extraction Mode"=0, "Edge Threshold"=75, "Edge Filter Size"=1, "Min Length"=25, "Row Search Step Size"=15, "Col Search Step Size"=15, "Max Endpoint Gap"=10, "Closed"=FALSE, "Subpixel"=FALSE}, " score"=500.0} ("SetParameter")) -> (data=w99:T19)  [unwired: 2 in, 1 out]
        n40 = call "GetShpaeResultValue.vi"("data"=w98, "SetParameter"=w99) -> ("ResultValues"=w97:string[])  [unwired: 8 in, 1 out]
      }
      frame 12 {
        n41 = Variant To Data(type="", Variant=w104) -> (data=w102:string)  [unwired: 1 in, 1 out]
        n42 = Build Array(w102) -> (w101:string[])
      }
      frame 13 {
        n43 = Variant To Data(type=T20 {"Points (pixel)"=[], "Points (real)"=[], "Length (pixel)"=0.0, "Length (real)"=0.0} ("ContourResult"), Variant=w108) -> (data=w107:T20, error out=w106:errorcluster)  [unwired: 1 in]
        n44 = call <vilib>:"Clear Errors.vi"("error in (no error)"=w106) -> ()  [unwired: 5 in, 2 out]
        n45 = call "GetContourResultValue.vi"("ContourResult"=w107) -> ("ContourResultValue"=w105:string[])  [unwired: 10 in]
      }
      frame 14 {
        n46 = Variant To Data(type=T21 {"Match Flag"=[], "Match Score"=[], "ROI Descriptor"={"Global Rectangle"=[], "Contours"=[]}} ("output cluster"), Variant=w116) -> (data=w113:T21, error out=w115:errorcluster)  [unwired: 1 in]
        n47 = call <vilib>:"Clear Errors.vi"("error in (no error)"=w115) -> ()  [unwired: 5 in, 2 out]
        n48 = Unbundle By Name(w113) -> ("Match Flag"=w112:bool[], "Match Score"=w111:i32[])
        n49 = for {
          tunnel: w112 -> [w123] mode=indexing
          tunnel: w111 -> [w120] mode=indexing
          tunnel: [w117] -> w110 mode=concatenating
          n50 = Number To Decimal String(number=w120) -> (decimal integer string=w118:string)  [unwired: 1 in]
          n51 = Select(t="TRUE", s=w123, f="FALSE") -> (s? t:f=w119:string)
          n52 = Build Array(w119, w118) -> (w117:string[])
        }
      }
    }
    n53 = Build Array (concatenate)(w8, w6) -> (w7:string[])
  }
  "TableValues" <- w1
